vi "Create Stop Event.vi"(8 "error in (no error)":errorcluster) -> (0 "error out":errorcluster, 3 "Stop Event out":refnum<user-event>)   [LabVIEW 2016, in "Stop Event.lvlib"]
uses:
  Stop Event.lvlib
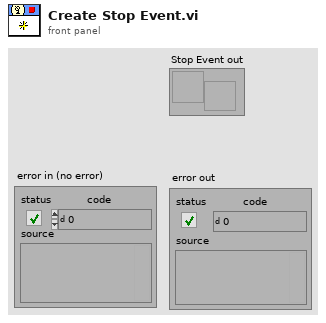
[diagram p1: front panel]
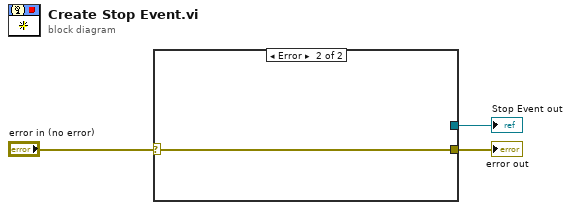
[diagram p0: block diagram]
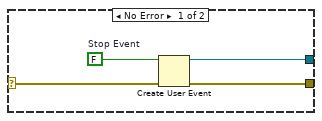
[diagram p2: hidden frame]
diagram:
  n1 = case shown="Error" "error in (no error)" {
    selector: "error in (no error)" -> [w7 w8]
    tunnel: [w6 w8] -> w2
    tunnel: [w4 _] -> w1
    frame No Error {
      w5 = FALSE  # Stop Event
      n2 = Create User Event(user event datatype=w5, error in=w7) -> (user event=w4:refnum<user-event>, error out=w6:errorcluster)
    }
    frame Error {
    }
  }
  "error out" <- w2
  "Stop Event out" <- w1
